vi "Control Panel.vi"(8 "error in (no error)":errorcluster, 11 "Fluke Calibrator in":refnum<class "Fluke Calibrator.lvclass">) -> (0 "error out":errorcluster, 3 "Fluke Calibrator out":refnum<class "Fluke Calibrator.lvclass">)   [LabVIEW 2012, in "Fluke Calibrator.lvclass"]
doc: "(Dynamic) A user-level application that simulates the physical front panel of the Instrument. Provide the user with buttons to manually control features of the instrument, and provide indicators of its current state."
uses:
  Fluke Calibrator.lvclass
  Fluke Calibrator.lvclass/Fluke Calibrator.ctl
panel:
  in  "Constantly Set":bool
  in  "Read to control":bool
  in  "Reset":bool
  in  "stop":bool
  in  "On/off":bool
  in  "Voltage Set":dbl min=0.0 max=4.0 step=0.001 format="%.7g"
  out "Voltage":dbl format="%.7g"
  in  "Set":bool
  in  "Read":bool
  # "Do not go above 4 V,\ndo not go negative"
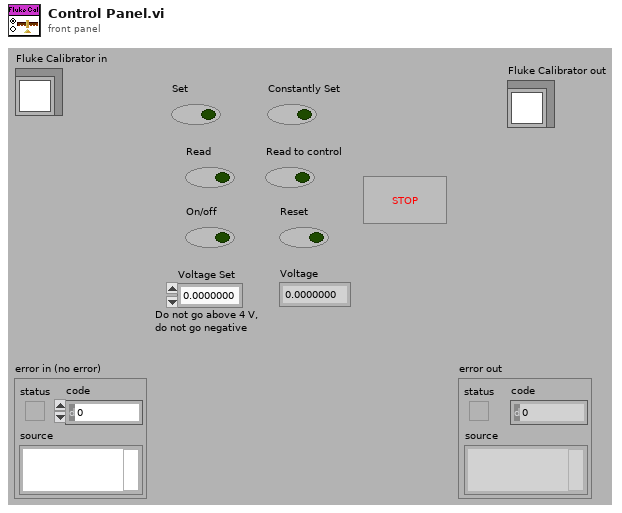
[diagram p1: front panel]
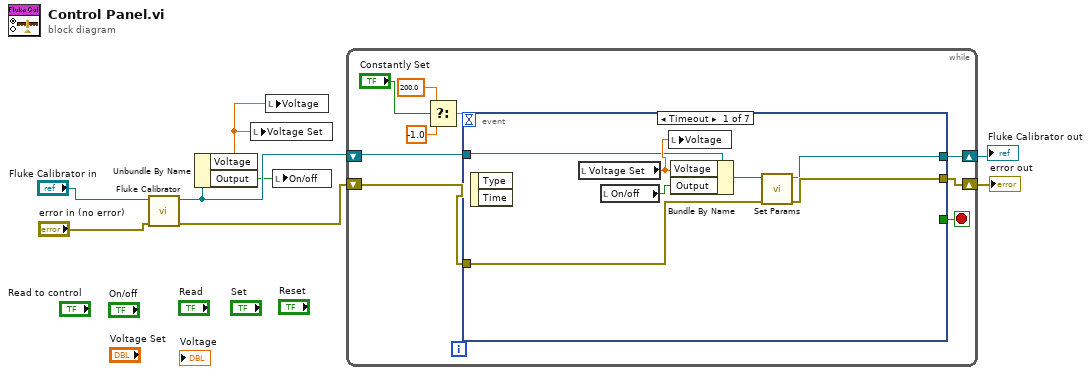
[diagram p0: block diagram]
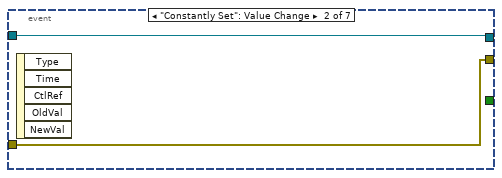
[diagram p2: hidden frame]
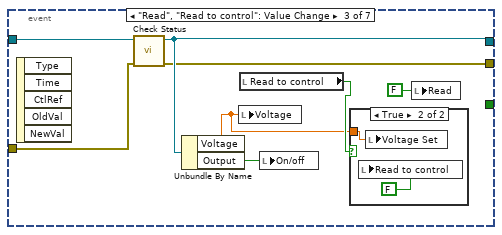
[diagram p3: hidden frame]
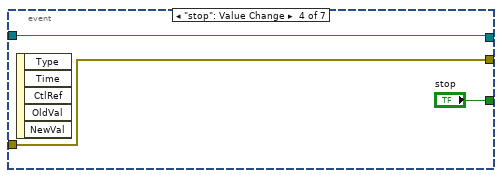
[diagram p5: hidden frame]
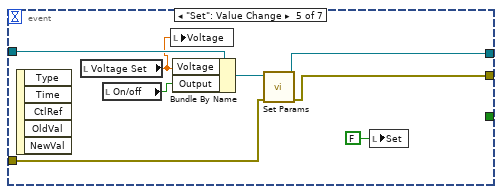
[diagram p6: hidden frame]
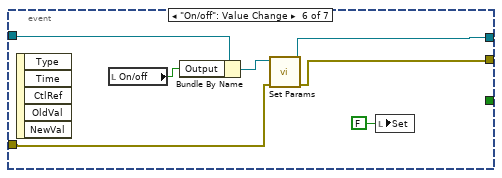
[diagram p7: hidden frame]
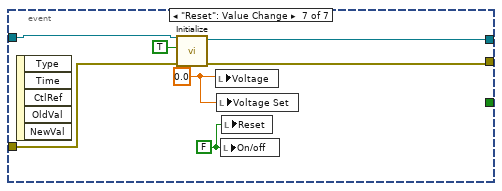
[diagram p8: hidden frame]
diagram:
  n1 = call "Fluke Calibrator.vi"("error in (no error)"="error in (no error)", "Fluke Calibrator in"="Fluke Calibrator in") -> ("error out"=w3:errorcluster, "Fluke Calibrator out"=w6:refnum<class "Fluke Calibrator.lvclass">)  [unwired: 8 in]
  n2 = Unbundle By Name(w6) -> ("Voltage"=w5:dbl, "Output"=w4:bool)
  n3 = local write "Voltage Set"(w5) -> ()
  n4 = local write "Voltage"(w5) -> ()
  n5 = local write "On/off"(w4) -> ()
  n6 = while {
    shift-right: [w15] -> w2
    shift-left: w6 -> [w17]
    shift-right: [w14] -> w1
    shift-left: w3 -> [w16]
    stop <- w13 stop-if-true
    n7 = Select(t=200.0, s="Constantly Set", f=-1.0) -> (s? t:f=w10:dbl)
    n8 = event shown="[0] Timeout" {
      selector: _ -> [_ _ _ _ _ _ _]
      dyn-events: _ -> [_ _ _ _ _ _ _]
      timeout: w10 -> [_ _ _ _ _ _ _]
      tunnel: w17 -> [w21 w26 w34 w38 w47 w51 w60]
      tunnel: w16 -> [w20 w25 w33 w37 w44 w50 w58]
      tunnel: [w18 w26 w31 w38 w42 w49 w59] -> w15
      tunnel: [w19 w25 w30 w37 w43 w48 w57] -> w14
      tunnel: [_ _ _ "stop" _ _ _] -> w13
      event Timeout {
        n9 = event-data() -> ()  [unwired: 1 in, 2 out]
        n10 = local read "Voltage Set"() -> (w22:dbl)
        n11 = local read "On/off"() -> (w24:bool)
        n12 = local write "Voltage"(w22) -> ()
        n13 = Bundle By Name(cluster=w21, "Voltage"=w22, "Output"=w24) -> (w23:refnum<class "Fluke Calibrator.lvclass">)
        n14 = call "Set Params.vi"("error in (no error)"=w20, "Fluke Calibrator in"=w23) -> ("error out"=w19:errorcluster, "Fluke Calibrator out"=w18:refnum<class "Fluke Calibrator.lvclass">)  [unwired: 8 in]
      }
      event "Constantly Set": Value Change {
        n15 = event-data() -> ()  [unwired: 1 in, 5 out]
      }
      event "Read", "Read to control": Value Change {
        n16 = event-data() -> ()  [unwired: 1 in, 5 out]
        n17 = call-dynamic "Check Status.vi"("error in (no error)"=w33, "Fluke Calibrator in"=w34) -> ("error out"=w30:errorcluster, "Fluke Calibrator out"=w31:refnum<class "Fluke Calibrator.lvclass">)  [unwired: 6 in, 2 out]
        n18 = Unbundle By Name(w31) -> ("Voltage"=w27:dbl, "Output"=w32:bool)
        n19 = local write "Voltage"(w27) -> ()
        n20 = local read "Read to control"() -> (w28:bool)
        n21 = local write "On/off"(w32) -> ()
        n22 = case shown="True" w28 {
          tunnel: w27 -> [_ w35]
          frame False {
          }
          frame True {
            n23 = local write "Read to control"(FALSE) -> ()
            n24 = local write "Voltage Set"(w35) -> ()
          }
        }
        n25 = local write "Read"(FALSE ("Read")) -> ()
      }
      event "stop": Value Change {
        n26 = event-data() -> ()  [unwired: 1 in, 5 out]
      }
      event "Set": Value Change {
        n27 = event-data() -> ()  [unwired: 1 in, 5 out]
        n28 = local read "Voltage Set"() -> (w41:dbl)
        n29 = local read "On/off"() -> (w46:bool)
        n30 = local write "Voltage"(w41) -> ()
        n31 = Bundle By Name(cluster=w47, "Voltage"=w41, "Output"=w46) -> (w45:refnum<class "Fluke Calibrator.lvclass">)
        n32 = call "Set Params.vi"("error in (no error)"=w44, "Fluke Calibrator in"=w45) -> ("error out"=w43:errorcluster, "Fluke Calibrator out"=w42:refnum<class "Fluke Calibrator.lvclass">)  [unwired: 8 in]
        n33 = local write "Set"(FALSE ("Set")) -> ()
      }
      event "On/off": Value Change {
        n34 = event-data() -> ()  [unwired: 1 in, 5 out]
        n35 = local read "On/off"() -> (w54:bool)
        n36 = Bundle By Name(cluster=w51, "Output"=w54) -> (w53:refnum<class "Fluke Calibrator.lvclass">)
        n37 = call "Set Params.vi"("error in (no error)"=w50, "Fluke Calibrator in"=w53) -> ("error out"=w48:errorcluster, "Fluke Calibrator out"=w49:refnum<class "Fluke Calibrator.lvclass">)  [unwired: 8 in]
        n38 = local write "Set"(FALSE ("Set")) -> ()
      }
      event "Reset": Value Change {
        w56 = FALSE ("On/off")
        w55 = 0.0 ("Voltage")
        n39 = event-data() -> ()  [unwired: 1 in, 5 out]
        n40 = call "Initialize.vi"("error in (no error)"=w58, "Reset?"=TRUE, "Fluke Calibrator in"=w60) -> ("error out"=w57:errorcluster, "Fluke Calibrator out"=w59:refnum<class "Fluke Calibrator.lvclass">)  [unwired: 7 in]
        n41 = local write "Voltage"(w55) -> ()
        n42 = local write "Voltage Set"(w55) -> ()
        n43 = local write "On/off"(w56) -> ()
        n44 = local write "Reset"(w56) -> ()
      }
    }
  }
  "error out" <- w1
  "Fluke Calibrator out" <- w2
